vi "GlobalGetSetMeasurementTimings.vi"() -> ()   [LabVIEW 2011]
panel:
  in  "Measurement Duration":dbl
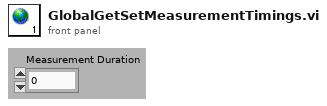
[diagram p1: front panel]
diagram:
